vi "Item_OnCommand.vi"(10 "Command ID":string, 11 "Object":T1) -> ()   [LabVIEW 2020, in "Project Provider.lvlib"]
uses:
  Project Provider.lvlib
  <resource>/Framework/Providers/API/ItemRef.ctl
panel:
  out "error out":errorcluster
  in  "error in":errorcluster
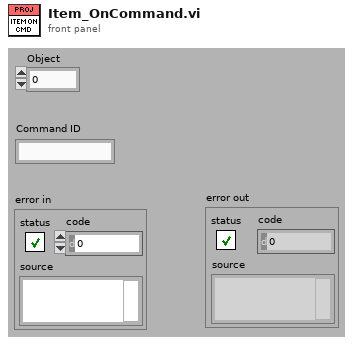
[diagram p1: front panel]
types:
  T1 = typedef "ItemRef.ctl" = u64
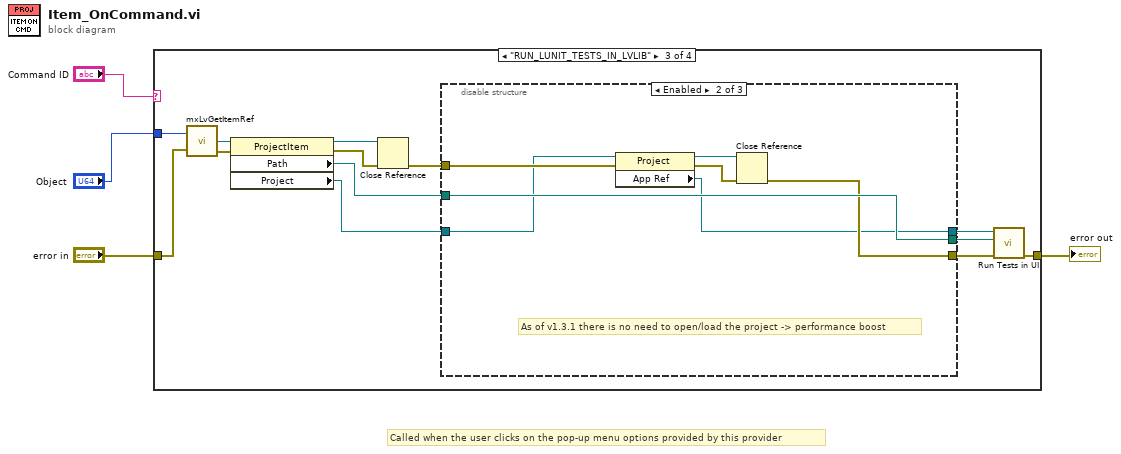
[diagram p0: block diagram]
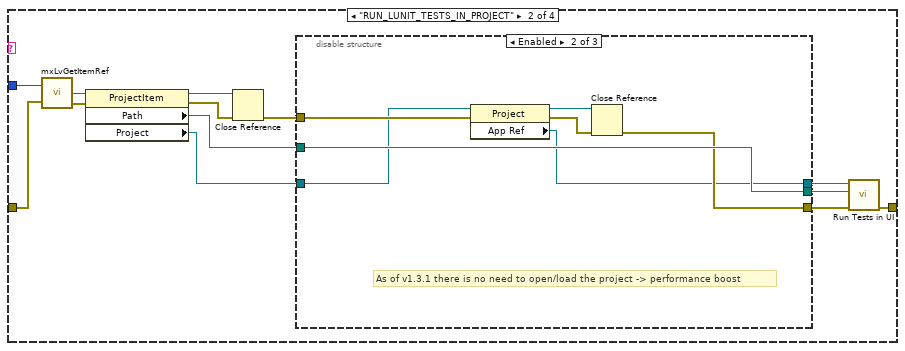
[diagram p3: hidden frame]
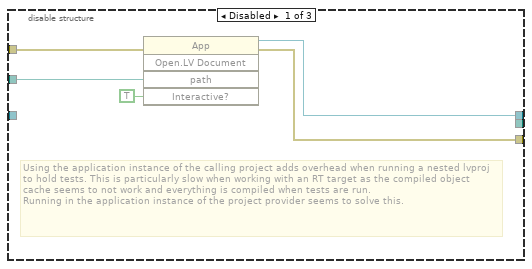
[diagram p4: hidden frame]
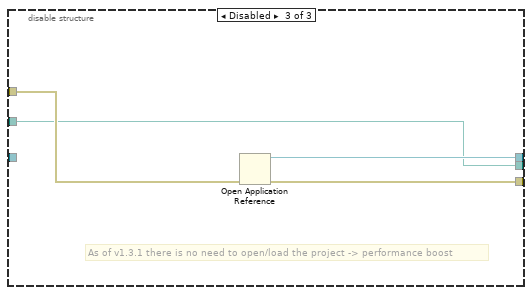
[diagram p5: hidden frame]
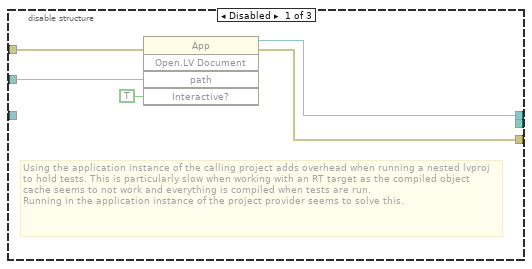
[diagram p6: hidden frame]
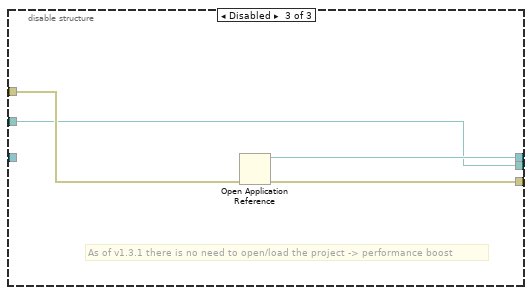
[diagram p7: hidden frame]
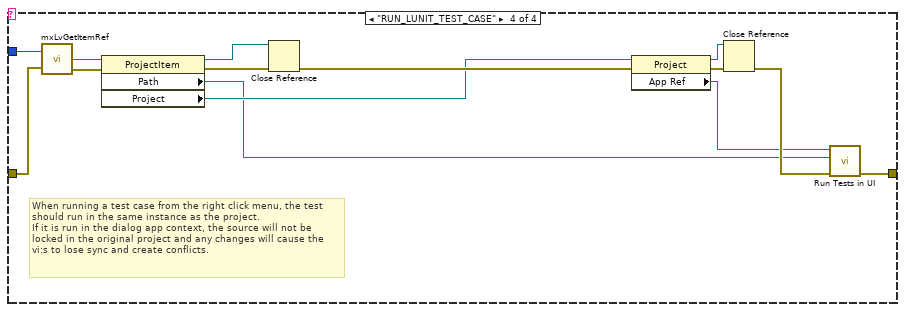
[diagram p8: hidden frame]
diagram:
  # "Called when the user clicks on the pop-up menu options provided by this provider"
  n1 = case shown="\"RUN_LUNIT_TESTS_IN_LVLIB\"" "Command ID" {
    tunnel: "error in" -> [w5 w17 w46 w76]
    tunnel: [w5 w11 w40 w71] -> w2
    tunnel: "Object" -> [_ w18 w47 w77]
    frame Default {
    }
    frame "RUN_LUNIT_TESTS_IN_PROJECT" {
      n2 = call <resource>:"mxLvGetItemRef.vi"("Item"=w18, "error in"=w17) -> ("Item Refnum"=w16:refnum<vi>, "error out"=w13:errorcluster)  [unwired: 1 out]
      n3 = property class="ProjectItem"(reference=w16, error in=w13) -> (reference out=w14:refnum<vi>, error out=w15:errorcluster, "Path"=w9:path, "Project"=w6:refnum<vi>)
      n4 = Close Reference(reference=w14, error in (no error)=w15) -> (error out=w12:errorcluster)
      n5 = disable-structure shown="Enabled" {
        disable-tunnel: w12 -> [w23 w27 w32]
        disable-tunnel: [w22 w26 w33] -> w10
        disable-tunnel: w9 -> [w21 w30 w31]
        disable-tunnel: [w19 w24 w34] -> w8
        disable-tunnel: [_ w30 w31] -> w7
        disable-tunnel: w6 -> [_ w25 _]
        frame Disabled {
          # "Using the application instance of the calling project adds overhead when running a nested lvproj to hold tests. This is particularly slow when working with an RT target as the compiled object cache seems to not work and everything is compiled when tests are run.\nRunning in the application instance of the project provider seems to solve this."
          n6 = invoke class="App" method="Open.LV Document"(error in=w23, "path"=w21, "Interactive?"=TRUE) -> (reference out=w19:refnum<vi>, error out=w22:errorcluster)  [unwired: 2 in, 3 out]
        }
        frame Enabled {
          # "As of v1.3.1 there is no need to open/load the project -> performance boost"
          n7 = property class="Project"(reference=w25, error in=w27) -> (reference out=w29:refnum<vi>, error out=w28:errorcluster, "App Ref"=w24:refnum<vi>)
          n8 = Close Reference(reference=w29, error in (no error)=w28) -> (error out=w26:errorcluster)
        }
        frame Disabled {
          # "As of v1.3.1 there is no need to open/load the project -> performance boost"
          n9 = Open Application Reference(8:w32) -> (0:w33:errorcluster, 3:w34:refnum<vi>)  [unwired: 3 in]
        }
      }
      n10 = call "Run Tests in UI.vi"("error in (no error)"=w10, "Path"=w7, "Application"=w8) -> ("error out"=w11:errorcluster)  [unwired: 8 in]
    }
    frame "RUN_LUNIT_TESTS_IN_LVLIB" {
      n11 = call <resource>:"mxLvGetItemRef.vi"("Item"=w47, "error in"=w46) -> ("Item Refnum"=w45:refnum<vi>, "error out"=w42:errorcluster)  [unwired: 1 out]
      n12 = property class="ProjectItem"(reference=w45, error in=w42) -> (reference out=w43:refnum<vi>, error out=w44:errorcluster, "Path"=w38:path, "Project"=w35:refnum<vi>)
      n13 = Close Reference(reference=w43, error in (no error)=w44) -> (error out=w41:errorcluster)
      n14 = disable-structure shown="Enabled" {
        disable-tunnel: w41 -> [w52 w56 w61]
        disable-tunnel: [w51 w55 w62] -> w39
        disable-tunnel: w38 -> [w50 w59 w60]
        disable-tunnel: [w48 w53 w63] -> w37
        disable-tunnel: [_ w59 w60] -> w36
        disable-tunnel: w35 -> [_ w54 _]
        frame Disabled {
          # "Using the application instance of the calling project adds overhead when running a nested lvproj to hold tests. This is particularly slow when working with an RT target as the compiled object cache seems to not work and everything is compiled when tests are run.\nRunning in the application instance of the project provider seems to solve this."
          n15 = invoke class="App" method="Open.LV Document"(error in=w52, "path"=w50, "Interactive?"=TRUE) -> (reference out=w48:refnum<vi>, error out=w51:errorcluster)  [unwired: 2 in, 3 out]
        }
        frame Enabled {
          # "As of v1.3.1 there is no need to open/load the project -> performance boost"
          n16 = property class="Project"(reference=w54, error in=w56) -> (reference out=w58:refnum<vi>, error out=w57:errorcluster, "App Ref"=w53:refnum<vi>)
          n17 = Close Reference(reference=w58, error in (no error)=w57) -> (error out=w55:errorcluster)
        }
        frame Disabled {
          # "As of v1.3.1 there is no need to open/load the project -> performance boost"
          n18 = Open Application Reference(8:w61) -> (0:w62:errorcluster, 3:w63:refnum<vi>)  [unwired: 3 in]
        }
      }
      n19 = call "Run Tests in UI.vi"("error in (no error)"=w39, "Path"=w36, "Application"=w37) -> ("error out"=w40:errorcluster)  [unwired: 8 in]
    }
    frame "RUN_LUNIT_TEST_CASE" {
      # "When running a test case from the right click menu, the test should run in the same instance as the project.\nIf it is run in the dialog app context, the source will not be locked in the original project and any changes will cause the vi:s to lose sync and create conflicts."
      n20 = call <resource>:"mxLvGetItemRef.vi"("Item"=w77, "error in"=w76) -> ("Item Refnum"=w75:refnum<vi>, "error out"=w72:errorcluster)  [unwired: 1 out]
      n21 = property class="ProjectItem"(reference=w75, error in=w72) -> (reference out=w73:refnum<vi>, error out=w74:errorcluster, "Path"=w66:path, "Project"=w67:refnum<vi>)
      n22 = Close Reference(reference=w73, error in (no error)=w74) -> (error out=w69:errorcluster)
      n23 = property class="Project"(reference=w67, error in=w69) -> (reference out=w65:refnum<vi>, error out=w64:errorcluster, "App Ref"=w68:refnum<vi>)
      n24 = Close Reference(reference=w65, error in (no error)=w64) -> (error out=w70:errorcluster)
      n25 = call "Run Tests in UI.vi"("error in (no error)"=w70, "Path"=w66, "Application"=w68) -> ("error out"=w71:errorcluster)  [unwired: 8 in]
    }
  }
  "error out" <- w2
